vi "test_RS-xxx to GPIB ConvBox Initialize.vi"(8 "error in (no error)":errorcluster, 11 "TestCase in":refnum<class "Instrument Addon Serial Protocols Unit Tests.lvclass">) -> (0 "error out":errorcluster, 3 "TestCase out":refnum<class "Instrument Addon Serial Protocols Unit Tests.lvclass">)   [LabVIEW 2023, in "Instrument Addon Serial Protocols Unit Tests.lvclass"]
uses:
  Instrument Addon Serial Protocols Unit Tests.lvclass
  <vilib>/addons/_JKI Toolkits/VI Tester/TestCase.llb/TestCase.lvclass
  Listener/ListenerClassControls/Operation.ctl
  Listener/Listener.lvclass
  RS-xxx to GPIB ConvBox/RS-xxx to GPIB ConvBox.lvclass
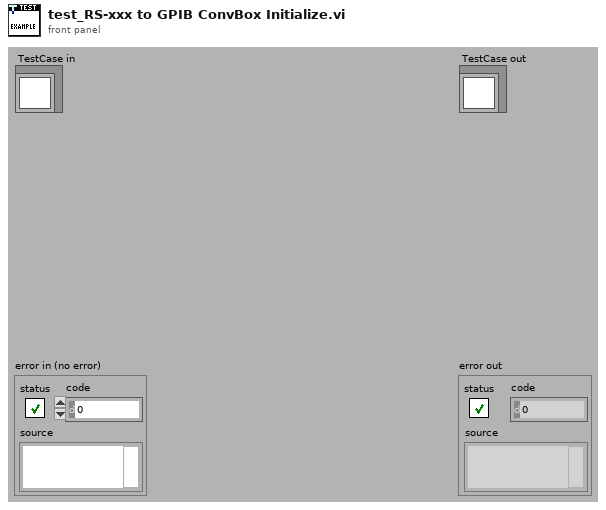
[diagram p1: front panel]
types:
  T1 = cluster{"IST bit sense":bool, "System controller":bool, "Assert Ren with IFC":bool}[]
  T2 = typedef "Listener.lvclass/Operation.ctl" = enum16{"Read", "Write"}
  T3 = typedef "Listener.lvclass/RS-xxx To GPIB ConvBox Data Structure.ctl" = cluster{"Data":string, "Command Messages Read":string[], "Address":string, "Data Length":u32}
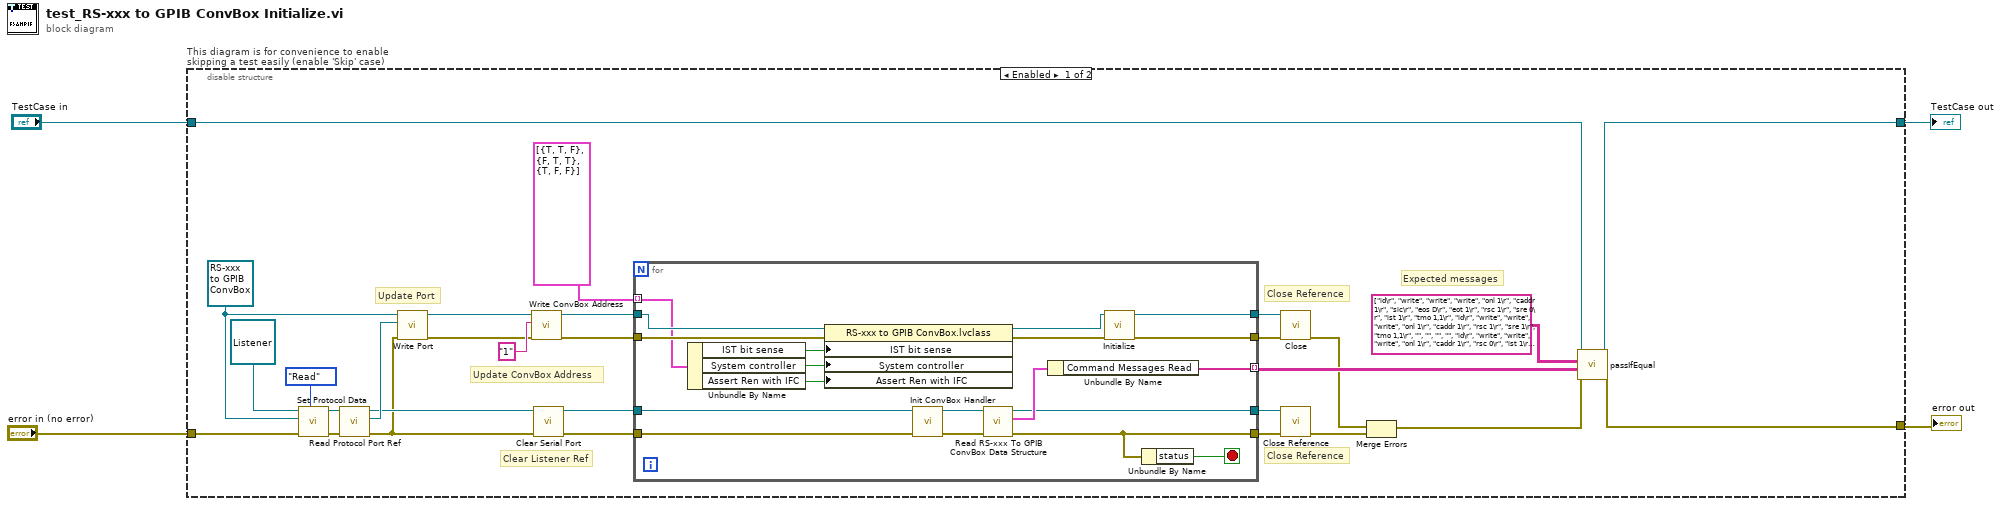
[diagram p0: block diagram]
diagram:
  n1 = disable-structure "This diagram is for convenience to enable skipping a test easily (enable 'Skip' case)" shown="Enabled" {
    disable-tunnel: "TestCase in" -> [w33 w56]
    disable-tunnel: [w32 w54] -> w1
    disable-tunnel: [w11 w55] -> w3
    disable-tunnel: "error in (no error)" -> [w31 w53]
    frame Enabled {
      w18 = refnum<class "RS-xxx to GPIB ConvBox.lvclass"> refnum ("Protocols.lvlib:RS-xxx to GPIB ConvBox.lvclass")
      # "Close Reference"
      # "Close Reference"
      # "Update Port"
      # "Expected messages"
      # "Update ConvBox Address"
      # "Clear Listener Ref"
      n2 = call "Set Protocol Data.vi"("Operation"=Operation."Read", "error in (no error)"=w31, "Protocols.lvlib:Protocol Parent.lvclass"=w18, "Listener In.lvclass"=refnum<class "Listener.lvclass"> refnum ("Listener.lvclass")) -> ("error out"=w22:errorcluster, "Listener Out.lvclass"=w21:refnum<class "Listener.lvclass">)  [unwired: 6 in]
      n3 = call "Read Protocol Port Ref.vi"("error in (no error)"=w22, "Listener in"=w21) -> ("error out"=w15:errorcluster, "Protocol Port Ref"=w17:refnum<visa-resource-name>, "Listener out"=w16:refnum<class "Listener.lvclass">)  [unwired: 7 in]
      n4 = call "Write Port.vi"("error in (no error)"=w15, "Port"=w17, "RS232 to GPIB ConvBox in"=w18) -> ("error out"=w20:errorcluster, "RS232 to GPIB ConvBox out"=w19:refnum<class "RS-xxx to GPIB ConvBox.lvclass">)  [unwired: 7 in]
      n5 = call "Write ConvBox Address.vi"("error in (no error)"=w20, "ConvBox Address"="1", "RS232 to GPIB ConvBox in"=w19) -> ("error out"=w28:errorcluster, "RS232 to GPIB ConvBox out"=w27:refnum<class "RS-xxx to GPIB ConvBox.lvclass">)  [unwired: 7 in]
      n6 = call "Clear Serial Port.vi"("error in (no error)"=w15, "Listener In.lvclass"=w16) -> ("error out"=w25:errorcluster, "Listener out"=w24:refnum<class "Listener.lvclass">)  [unwired: 8 in]
      n7 = for {
        tunnel: w27 -> [w39]
        tunnel: w24 -> [w51]
        tunnel: w25 -> [w52]
        tunnel: [w46] -> w9
        tunnel: w28 -> [w41]
        tunnel: [w50] -> w7
        tunnel: [w44] -> w12 mode=indexing
        tunnel: [w43] -> w6
        tunnel: [w42] -> w10
        tunnel: T1 [{"IST bit sense"=TRUE, "System controller"=TRUE, "Assert Ren with IFC"=FALSE}, {"IST bit sense"=FALSE, "System controller"=TRUE, "Assert Ren with IFC"=TRUE}, {"IST bit sense"=TRUE, "System controller"=FALSE, "Assert Ren with IFC"=FALSE}] -> [w37] mode=indexing
        stop <- w45 stop-if-true
        n8 = Unbundle By Name(w37) -> ("IST bit sense"=w36:bool, "System controller"=w35:bool, "Assert Ren with IFC"=w34:bool)
        n9 = property class="RS-xxx to GPIB ConvBox.lvclass"(reference=w39, error in=w41, "IST bit sense"=w36, "System controller"=w35, "Assert Ren with IFC"=w34) -> (reference out=w38:refnum<class "RS-xxx to GPIB ConvBox.lvclass">, error out=w40:errorcluster)
        n10 = call "Init ConvBox Handler.vi"("error in (no error)"=w52, "Listener in"=w51) -> ("error out"=w49:errorcluster, "Listener out"=w48:refnum<class "Listener.lvclass">)  [unwired: 8 in]
        n11 = call-dynamic "Read RS-xxx To GPIB ConvBox Data Structure.vi"("error in (no error)"=w49, "Listener in"=w48) -> ("error out"=w46:errorcluster, "RS-xxx To GPIB ConvBox Data Structure"=w47:T3, "Listener out"=w42:refnum<class "Listener.lvclass">)  [unwired: 7 in]
        n12 = Unbundle By Name(w47) -> ("Command Messages Read"=w44:string[])
        n13 = call-dynamic "Initialize.vi"("error in (no error)"=w40, "RS232 to GPIB ConvBox in"=w38) -> ("error out"=w50:errorcluster, "RS232 to GPIB ConvBox out"=w43:refnum<class "RS-xxx to GPIB ConvBox.lvclass">)  [unwired: 8 in]
        n14 = Unbundle By Name(w46) -> ("status"=w45:bool)
      }
      n15 = call-dynamic "Close.vi"("error in (no error)"=w7, "RS232 to GPIB ConvBox in"=w6) -> ("error out"=w5:errorcluster)  [unwired: 8 in, 1 out]
      n16 = call "Close Reference.vi"("error in (no error)"=w9, "Listener In.lvclass"=w10) -> ("error out"=w8:errorcluster)  [unwired: 8 in, 1 out]
      n17 = Merge Errors(w5, w8) -> (w23:errorcluster)
      n18 = call-dynamic "passIfEqual.vi"("error in (no error)"=w23, "y"=w12, "x"=string[][] [["id\r", "write", "write", "write", "onl 1\r", "caddr 1\r", "sic\r", "eos D\r", "eot 1\r", "rsc 1\r", "sre 0\r", "ist 1\r", "tmo 1,1\r"], ["id\r", "write", "write", "write", "onl 1\r", "caddr 1\r", "rsc 1\r", "sre 1\r", "tmo 1,1\r", "", "", "", ""], ["id\r", "write", "write", "write", "onl 1\r", "caddr 1\r", "rsc 0\r", "ist 1\r", "tmo 1,1\r", "", "", "", ""]] ("Command Messages Read"), "TestCase in"=w33) -> ("error out"=w11:errorcluster, "TestCase out"=w32:refnum<class "Instrument Addon Serial Protocols Unit Tests.lvclass">)  [unwired: 6 in]
    }
    frame Disabled {
      # "skip test result while test is under development"
      n19 = call <vilib>:"skip.vi"("error in (no error)"=w53, "TestCase in"=w56) -> ("error out"=w55:errorcluster, "TestCase out"=w54:refnum<class "Instrument Addon Serial Protocols Unit Tests.lvclass">)  [unwired: 8 in]
    }
  }
  "error out" <- w3
  "TestCase out" <- w1
